vi "PipBoy_Cmd-Next.vi"(8 "error in (no error)":errorcluster, 11 "DataIn":T1) -> (0 "error out":errorcluster, 3 "DataOut":T1)   [LabVIEW 2014]
uses:
  ctls/PipBoy_PipBoyData.ctl
  ctls/PipBoy_ProcComm.ctl
  System.Windows.Forms
  ctls/PipBoy_PipBoyCommand.ctl
  ctls/PipBoy_Message.ctl
  modules/support/Message Queue/All Message Queues.ctl
  modules/support/Message Queue/Message Cluster.ctl
  ctls/PipBoy_FileConf.ctl
  ctls/PipBoy_PicComm.ctl
  ctls/PipBoy_GeneralParams.ctl
  ctls/PipBoy_Pages.ctl
  modules/support/Message Queue/Message Queue.lvlib
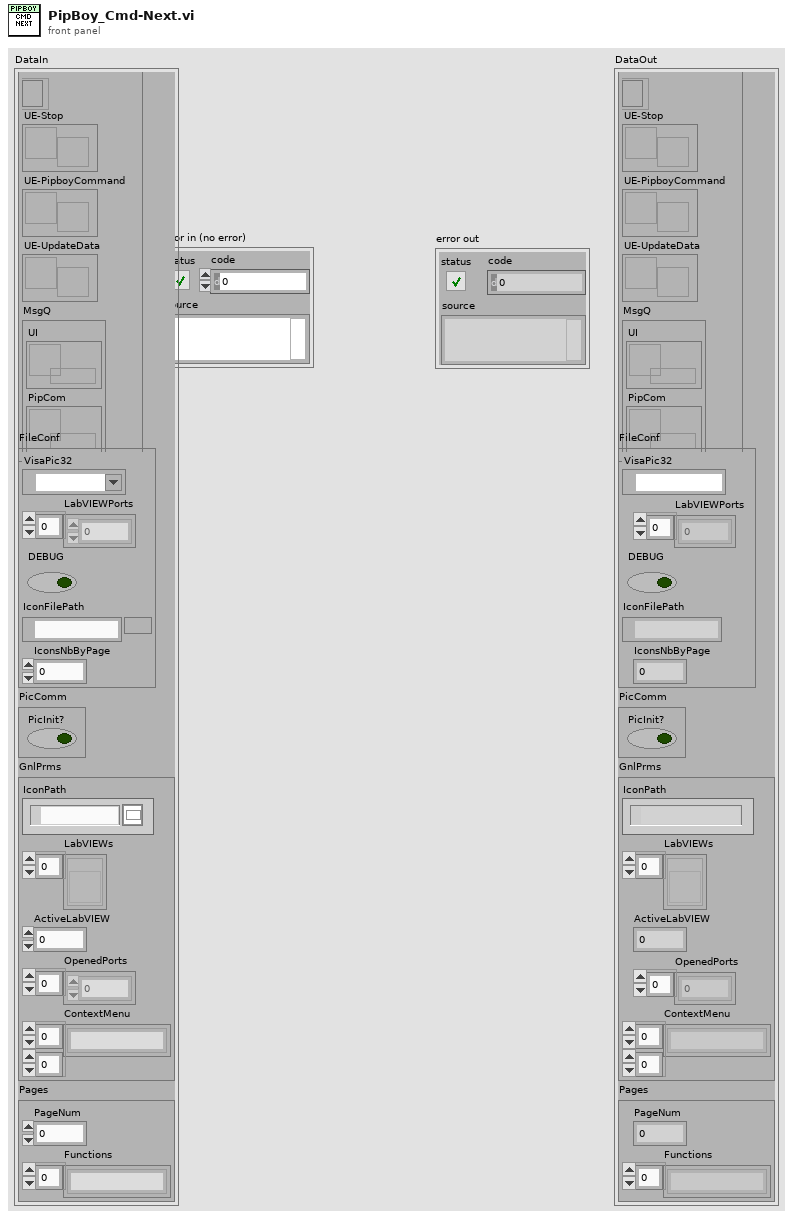
[diagram p1: front panel]
types:
  T1 = typedef "PipBoy_PipBoyData.ctl" = cluster{"ProcComm":T2, "FileConf":T4, "PicComm":T5, "GnlPrms":T6, "Pages":T7}
  T2 = typedef "PipBoy_ProcComm.ctl" = cluster{"NotifyIconRef":refnum<k24>, "UE-Stop":refnum<user-event>, "UE-PipboyCommand":refnum<user-event>, "UE-UpdateData":refnum<user-event>, "MsgQ":T3}
  T3 = typedef "Message Queue.lvlib/All Message Queues.ctl" = cluster{"UI":refnum<queue>, "PipCom":refnum<queue>}
  T4 = typedef "PipBoy_FileConf.ctl" = cluster{"VisaPic32":refnum<visa-resource-name>, "LabVIEWPorts":u16[], "DEBUG":bool, "IconFilePath":path, "IconsNbByPage":i32}
  T5 = typedef "PipBoy_PicComm.ctl" = cluster{"PicInit?":bool}
  T6 = typedef "PipBoy_GeneralParams.ctl" = cluster{"IconPath":path, "LabVIEWs":refnum<vi>[], "ActiveLabVIEW":i32, "OpenedPorts":u16[], "ContextMenu":string[][]}
  T7 = typedef "PipBoy_Pages.ctl" = cluster{"PageNum":i32, "Functions":string[]}
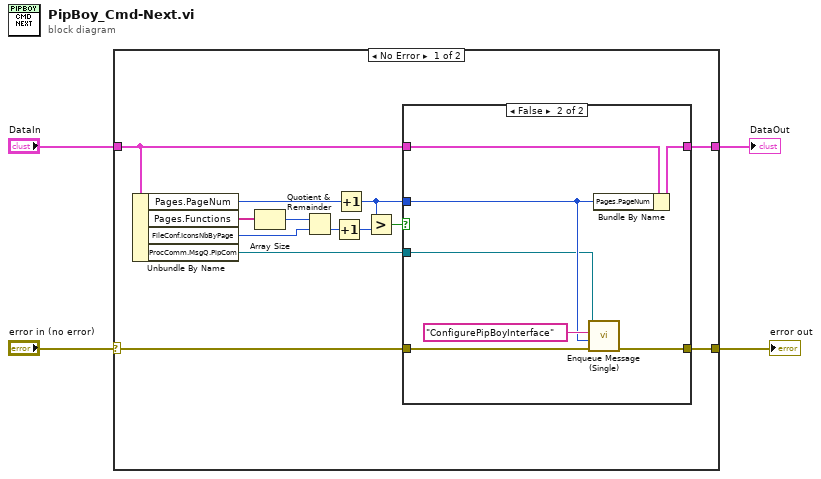
[diagram p0: block diagram]
diagram:
  n1 = case shown="No Error" "error in (no error)" {
    selector: "error in (no error)" -> [w17 w28]
    tunnel: [w16 w28] -> w4
    tunnel: "DataIn" -> [w15 w27]
    tunnel: [w14 w27] -> w1
    frame No Error {
      n2 = Unbundle By Name(w15) -> ("Pages.PageNum"=w11:i32, "Pages.Functions"=w5:string[], "FileConf.IconsNbByPage"=w13:i32, "ProcComm.MsgQ.PipCom"=w6:refnum<queue>)
      n3 = Array Size(array=w5) -> (size(s)=w8:i32)
      n4 = Quotient & Remainder(x=w8, y=w13) -> (floor(x/y)=w7:i32)  [unwired: 1 out]
      n5 = Increment(x=w7) -> (x+1=w12:i32)
      n6 = Increment(x=w11) -> (x+1=w9:i32)
      n7 = Greater?(x=w9, y=w12) -> (0:w10:bool)
      n8 = case shown="False" w10 {
        tunnel: w17 -> [w19 w25]
        tunnel: [w19 w24] -> w16
        tunnel: w15 -> [w18 w23]
        tunnel: [w18 w22] -> w14
        tunnel: w9 -> [_ w21]
        tunnel: w6 -> [_ w20]
        frame True {
        }
        frame False {
          n9 = call "Enqueue Message (Single).vi"("error in (no error)"=w25, "Message Data"=w21, "Message"="ConfigurePipBoyInterface", "Message Queue"=w20) -> ("error out"=w24:errorcluster)  [unwired: 6 in, 1 out]
          n10 = Bundle By Name(cluster=w23, "Pages.PageNum"=w21) -> (w22:T1)
        }
      }
    }
    frame Error {
    }
  }
  "error out" <- w4
  "DataOut" <- w1
